vi "initialize_data_log.vi"(7 "Overwrite?":bool, 8 "error in (no error)":errorcluster, 9 "Initialization Data":variant, 10 "Path":path, 11 "scan_hdf5_log in":refnum<class "scan_2d_hdf5_log.lvclass">) -> (0 "error out":errorcluster, 3 "scan_hdf5_log out":refnum<class "scan_2d_hdf5_log.lvclass">)   [LabVIEW 2015, in "scan_2d_hdf5_log.lvclass"]
uses:
  scan_2d_hdf5_log.lvclass
  scan_2d_log_data.ctl
  scan_2d_hdf5_log.lvclass/scan_2d_hdf5_log.ctl
  <vilib>/UPVI/lvhdf5/dataset.llb/LVH5D Operation.ctl
  <vilib>/UPVI/lvhdf5/file.llb/LVH5F Operation.ctl
  <vilib>/Utility/miscctls.llb/LVRectTypeDef.ctl
  <vilib>/UPVI/lvhdf5/group.llb/H5G_obj_t.ctl
  <vilib>/UPVI/lvhdf5/utility.llb/Select HDF5 Dialog.vi
  <vilib>/UPVI/lvhdf5/utility.llb/Select HDF5 Dialog (Object Only).vi
  <vilib>/UPVI/lvhdf5/dataset.llb/Simple H5Dwrite (Variant).vi
  <vilib>/UPVI/lvhdf5/dataset.llb/Simple H5Dwrite.xnode
  <vilib>/UPVI/lvhdf5/library.llb/HDF5 Ref.ctl
  Detector_Class/Picoquant/Hydraharp/hydraharp/hydraharp.lvclass
  <vilib>/UPVI/lvhdf5/file.llb/H5Fclose.vi
  <vilib>/UPVI/lvhdf5/identifier.llb/Not an HDF5 Refnum Constant.vi
  <vilib>/Utility/error.llb/Error Cluster From Error Code.vi
  <vilib>/UPVI/lvhdf5/dataset.llb/OpenCreateReplace Dataset by Element Type.vi
  <vilib>/UPVI/lvhdf5/dataspace.llb/H5Sselect_hyperslab.vi
  <vilib>/UPVI/lvhdf5/dataset.llb/H5Dwrite (Variant).vi
  <vilib>/UPVI/lvhdf5/dataset.llb/H5Dget_space.vi
  <vilib>/UPVI/lvhdf5/attribute.llb/private/LVH5AwriteWDTAttrs.vi
  <vilib>/UPVI/lvhdf5/dataspace.llb/H5Sclose.vi
  <vilib>/UPVI/lvhdf5/utility.llb/Select HDF5 Dialog (File and Object).vi
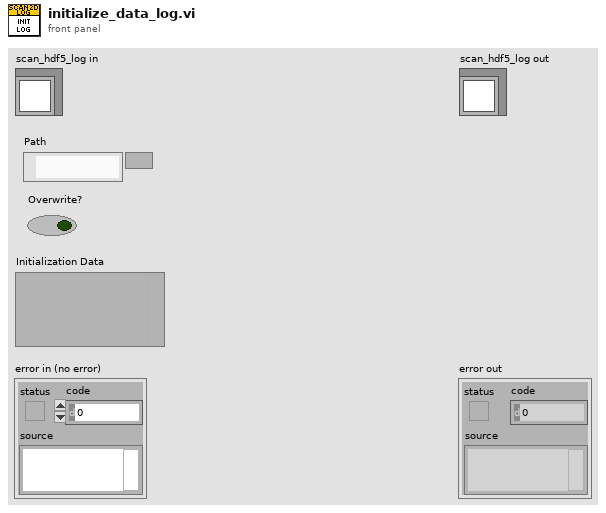
[diagram p1: front panel]
types:
  T1 = typedef "scan_2d_log_data.ctl" = cluster{"x_positions (mm)":dbl[], "y_positions":dbl[]}
  T2 = typedef "LVH5D Operation.ctl" = enum16{"open", "replace", "create", "open or create", "create or replace", "create or replace with confirmation"}
  T3 = typedef "LVRectTypeDef.ctl" = cluster{"Left":i16, "Top":i16, "Right":i16, "Bottom":i16}
  T4 = cluster{"Behavior":enum32{"Invalid", "Default", "Floating", "Floating/Auto-Hide", "Modal"}, "Position":T3, "Center":bool, "Title":string}
  T5 = typedef "LVH5F Operation.ctl" = enum16{"open", "open or create", "create or replace", "create or replace (with confirmation)", "create", "open (read only)"}
  T6 = typedef "H5G_obj_t.ctl" = i32
  T7 = cluster{"Object Types (any)":T6[], "Object Pattern":string}
  T8 = typedef "HDF5 Ref.ctl" = refnum<k1>
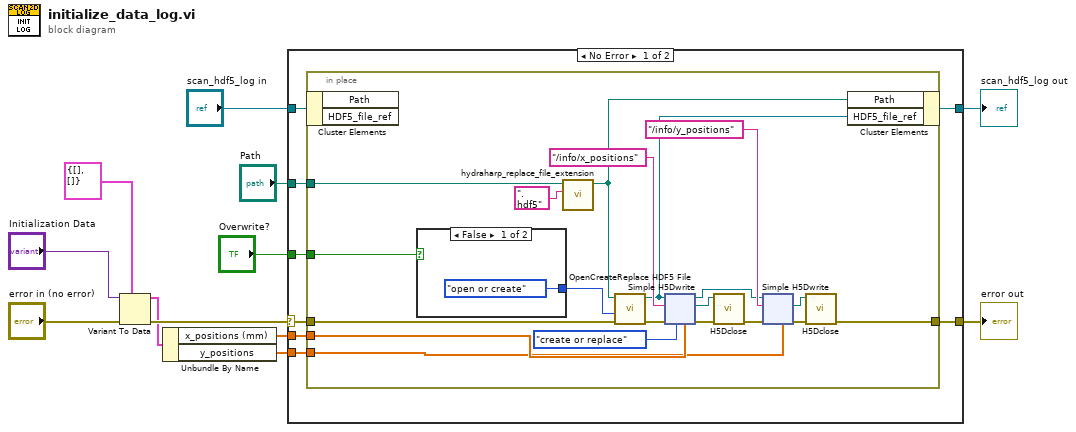
[diagram p0: block diagram]
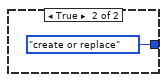
[diagram p2: hidden frame]
diagram:
  n1 = Variant To Data(error in="error in (no error)", type=T1 {"x_positions (mm)"=[], "y_positions"=[]} ("output cluster"), Variant="Initialization Data") -> (data=w4:T1, error out=w10:errorcluster)
  n2 = Unbundle By Name(w4) -> ("x_positions (mm)"=w2:dbl[], "y_positions"=w1:dbl[])
  n3 = case shown="No Error" w10 {
    selector: w10 -> [w18 w448]
    tunnel: "scan_hdf5_log in" -> [w20 w447]
    tunnel: "Overwrite?" -> [w19 _]
    tunnel: [w17 w447] -> w7
    tunnel: "Path" -> [w16 _]
    tunnel: [w15 w448] -> w5
    tunnel: w2 -> [w14 _]
    tunnel: w1 -> [w13 _]
    frame No Error {
      n4 = in-place {
        in-place-border: w19 -> [w37]
        in-place-border: w18 -> [w35]
        in-place-border: w16 -> [w32]
        in-place-border: [w21] -> w15
        in-place-border: w14 -> [w28]
        in-place-border: w13 -> [w25]
        n5 = in-place-cluster #1(w20) -> ()  [unwired: 2 out]
        n6 = case shown="False" w37 {
          tunnel: [LVH5F_Operation."open or create" ("function (open or create)") LVH5F_Operation."create or replace" ("function (open or create)")] -> w36
          frame False {
          }
          frame True {
          }
        }
        n7 = call "hydraharp_replace_file_extension.vi"("new_extension"=".hdf5", "input_file"=w32) -> ("new_name"=w33:path)  [unwired: 9 in]
        n8 = call <vilib>:"OpenCreateReplace HDF5 File.vi"("error in (no error)"=w35, "function (open or create)"=w36, "path"=w33) -> ("error out"=w34:errorcluster, "HDF5 Ref out"=w29:T8)  [unwired: 5 in]
        n9 = xnode "Simple H5Dwrite"("Dataset Path"="/info/x_positions", "error in (no error)"=w34, "operation (open or create)"=LVH5D_Operation."create or replace", "HDF5 Path or Ref"=w29, "Data"=w28) -> ("HDF5 Dataset Ref out"=w31:T8, "HDF5 Ref out"=w23:T8, "error out"=w30:errorcluster)  [unwired: 3 in]
        n10 = call <vilib>:"H5Dclose.vi"("error in (no error)"=w30, "HDF5 Dataset Ref"=w31) -> ("error out"=w22:errorcluster)  [unwired: 7 in]
        n11 = xnode "Simple H5Dwrite"("Dataset Path"="/info/y_positions", "error in (no error)"=w22, "HDF5 Path or Ref"=w23, "Data"=w25) -> ("HDF5 Dataset Ref out"=w27:T8, "error out"=w26:errorcluster)  [unwired: 4 in, 1 out]
        n12 = call <vilib>:"H5Dclose.vi"("error in (no error)"=w26, "HDF5 Dataset Ref"=w27) -> ("error out"=w21:errorcluster)  [unwired: 7 in]
        n13 = in-place-cluster #1("Path"=w33, "HDF5_file_ref"=w29) -> (w17:refnum<class "scan_2d_hdf5_log.lvclass">)
      }
    }
    frame Error {
    }
  }
  "error out" <- w5
  "scan_hdf5_log out" <- w7
